vi "PXI-Config Counter.vi"(0 "Sync Task":T1={"Task name"="AI01", "Task"="", "Dual-channel task?"=FALSE, "Regenerate?"=FALSE, "Clear?"=FALSE}, 11 "error in (no error)":errorcluster) -> (8 "Counter Task":T1={"Task name"="Counter", "Task"="", "Dual-channel task?"=FALSE, "Regenerate?"=FALSE, "Clear?"=FALSE}, 15 "error out":errorcluster)   [LabVIEW 2020]
uses:
  Type Defs/Task Struct.ctl
  PXI Globals.vi
  <vilib>/DAQmx/create/channels.llb/DAQmx Create Channel (CO-Pulse Generation-Ticks).vi
  <vilib>/DAQmx/configure/timing.llb/DAQmx Timing (Implicit).vi
  <vilib>/DAQmx/configure/trigger.llb/DAQmx Start Trigger (Digital Edge).vi
  <resource>/objmgr/daqmx.rc
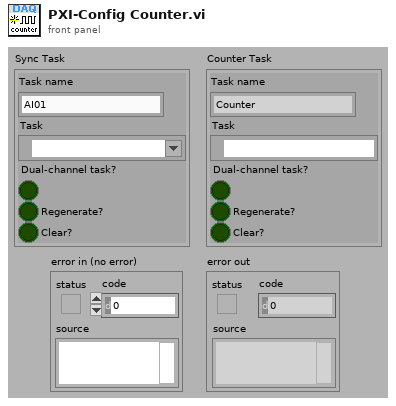
[diagram p1: front panel]
types:
  T1 = typedef "Task Struct.ctl" = cluster{"Task name":string, "Task":refnum<k21>, "Dual-channel task?":bool, "Regenerate?":bool, "Clear?":bool}
  T2 = typedef "Counter Params.ctl" = cluster{"Counter":tag, "Hi ticks":u32, "Low ticks":u32, "Idle state":i32, "Delay ticks":u32}
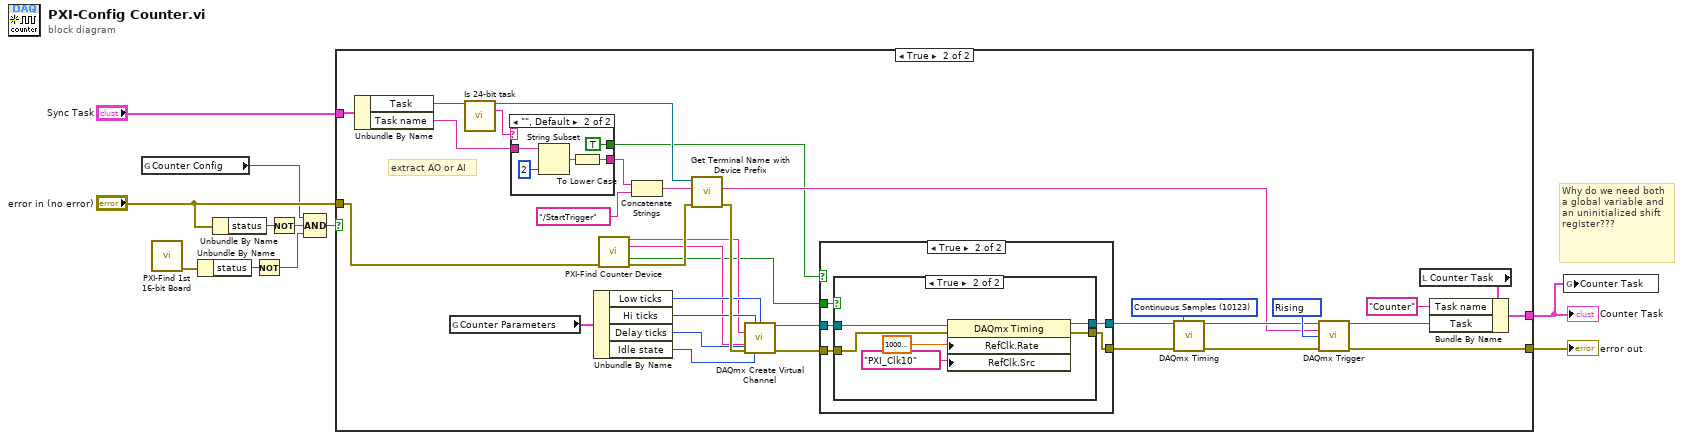
[diagram p0: block diagram]
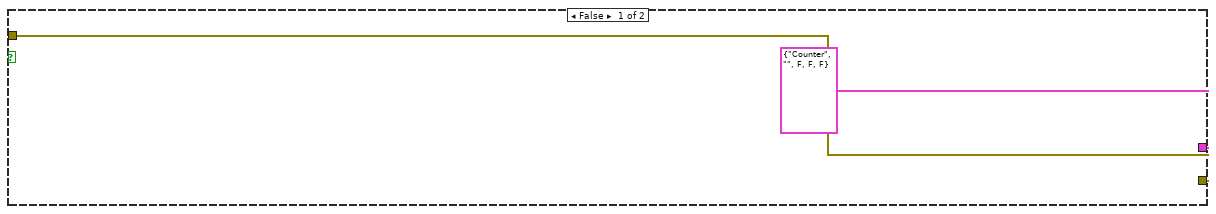
[diagram p2: hidden frame]
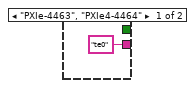
[diagram p5: hidden frame]
diagram:
  # "Why do we need both a global variable and an uninitialized shift register???"
  n1 = global read "PXI Globals.vi" "Counter Config"() -> (w5:bool)
  n2 = call "PXI-Find 1st 16-bit Board.vi"() -> ("error out"=w4:errorcluster)  [unwired: 9 in, 2 out]
  n3 = Unbundle By Name(w4) -> ("status"=w3:bool)
  n4 = Unbundle By Name("error in (no error)") -> ("status"=w7:bool)
  n5 = Not(x=w3) -> (.not. x?=w2:bool)
  n6 = Not(x=w7) -> (.not. x?=w8:bool)
  n7 = Compound Arithmetic op=AND(w5, w8, w2) -> (w1:bool)
  n8 = case shown="True" w1 {
    tunnel: [w12 w47] -> w11
    tunnel: "Sync Task" -> [_ w46]
    tunnel: [T1 {"Task name"="Counter", "Task"="", "Dual-channel task?"=FALSE, "Regenerate?"=FALSE, "Clear?"=FALSE} ("Counter Task") w45] -> w9
    tunnel: "error in (no error)" -> [w12 w22]
    frame False {
    }
    frame True {
      w43 = 10280 items=["Rising"=10280, "Falling"=10171] ("Trigger Edge")
      w44 = 10123 items=["Finite Samples"=10178, "Continuous Samples"=10123] ("sample mode")
      # "extract AO or AI"
      n9 = Unbundle By Name(w46) -> ("Task"=w18:refnum<k21>, "Task name"=w38:string)
      n10 = global read "PXI Globals.vi" "Counter Parameters"() -> (w27:T2)
      n11 = call "Is 24-bit task.vi"("task"=w18) -> ("task out"=w17:refnum<k21>, "Product Type"=w16:string)  [unwired: 9 in, 4 out]
      n12 = case shown="\"\", Default" w16 {
        tunnel: w38 -> [_ w67]
        tunnel: ["te0" w65] -> w32
        tunnel: [_ TRUE] -> w15
        frame "PXIe-4463", "PXIe4-4464" {
        }
        frame "", Default {
          n13 = String Subset(string=w67, length (rest)=2 ("length (rest)")) -> (substring=w66:string)  [unwired: 1 in]
          n14 = To Lower Case(string=w66) -> (all lower case string=w65:string)
        }
      }
      n15 = Unbundle By Name(w27) -> ("Low ticks"=w26:u32, "Hi ticks"=w25:u32, "Delay ticks"=w24:u32, "Idle state"=w23:i32)
      n16 = call "PXI-Find Counter Device.vi"("error in (no error)"=w22) -> ("Counter Channel"=w20:tag, "RefClk.Src"=w19:tag, "Is M-series board"=w14:bool, "error out"=w21:errorcluster)  [unwired: 10 in, 1 out]
      n17 = Concatenate Strings(w32, "/StartTrigger" ("Local Terminal Name")) -> (w39:string)
      n18 = call "Get Terminal Name with Device Prefix.vi"("error in (no error)"=w21, "Local Terminal Name"=w39, "task/channels in"=w17) -> ("error out"=w31:errorcluster, "Terminal Name with Device Prefix"=w33:string)  [unwired: 6 in, 1 out]
      n19 = call-poly <vilib>:"DAQmx Create Virtual Channel.vi"("high ticks"=w25, "low ticks"=w26, "counter"=w20, "source of ticks"=w19, "error in"=w31, "idle state"=w23, "initial delay"=w24) -> ("task out"=w29:refnum<k21>, "error out"=w30:errorcluster)  [unwired: 7 in]
      n20 = case shown="True" w15 {
        tunnel: [w49 w54] -> w37
        tunnel: [w48 w53] -> w36
        tunnel: w30 -> [w48 w52]
        tunnel: w29 -> [w49 w51]
        tunnel: w14 -> [_ w50]
        frame False {
        }
        frame True {
          n21 = case shown="True" w50 {
            tunnel: [w56 w62] -> w54
            tunnel: [w55 w61] -> w53
            tunnel: w52 -> [w55 w60]
            tunnel: w51 -> [w56 w59]
            frame False {
            }
            frame True {
              n22 = property class="DAQmx Timing"(reference=w59, error in=w60, "RefClk.Rate"=10000000.0, "RefClk.Src"=tag "PXI_Clk10") -> (reference out=w62:refnum<k21>, error out=w61:errorcluster)
            }
          }
        }
      }
      n23 = call-poly <vilib>:"DAQmx Timing.vi"("task/channels in"=w37, "sample mode"=w44, "error in"=w36) -> ("task out"=w35:refnum<k21>, "error out"=w34:errorcluster)  [unwired: 11 in]
      n24 = call-poly <vilib>:"DAQmx Trigger.vi"("task/channels in"=w35, "source"=w33, "edge"=w43, "error in"=w34) -> ("task out"=w41:refnum<k21>, "error out"=w47:errorcluster)  [unwired: 10 in]
      n25 = local read "Counter Task"() -> (w28:T1)
      n26 = Bundle By Name(cluster=w28, "Task name"="Counter" ("Channel"), "Task"=w41) -> (w45:T1)
    }
  }
  "error out" <- w11
  "Counter Task" <- w9
  n27 = global write "PXI Globals.vi" "Counter Task"(w9) -> ()
